vi "KH TURCK ETHERNETIP IOL Diagnostic.vi"(8 "Data_IO":T2, 11 "DataItem.Data":u8[](array[numeric])) -> (3 "Diagnostics":T1)   [LabVIEW 2021]
uses:
  KH TURCK ETHERNETIP TDef Enum IOL Data.ctl
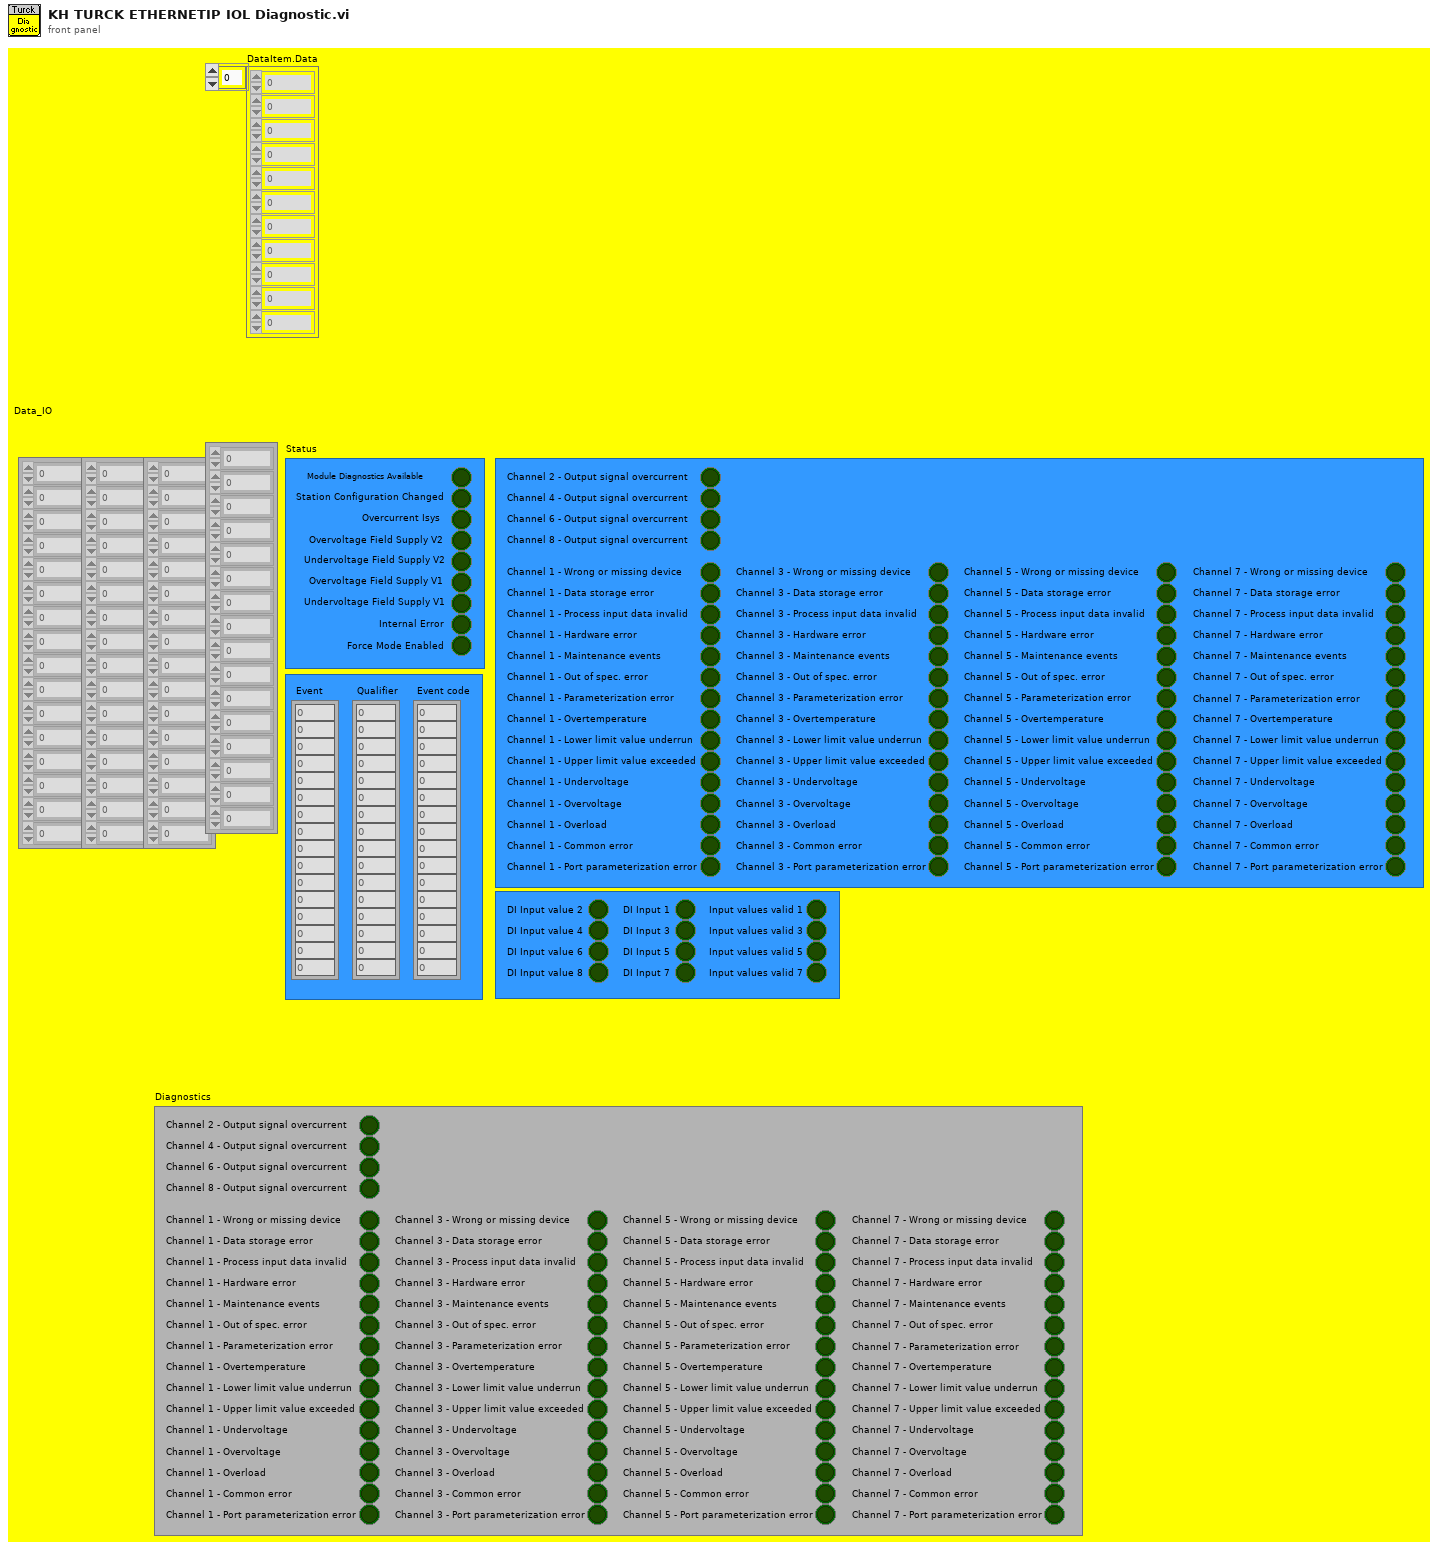
[diagram p1: front panel]
types:
  T1 = cluster{"Channel 2 - Output signal overcurrent":bool, "Channel 4 - Output signal overcurrent":bool, "Channel 6 - Output signal overcurrent":bool, "Channel 8 - Output signal overcurrent":bool, "Channel 1 - Wrong or missing device":bool, "Channel 3 - Wrong or missing device":bool, "Channel 5 - Wrong or missing device":bool, "Channel 7 - Wrong or missing device":bool, "Channel 1 - Data storage error":bool, "Channel 3 - Data storage error":bool, "Channel 5 - Data storage error":bool, "Channel 7 - Data storage error":bool, "Channel 1 - Process input data invalid":bool, "Channel 3 - Process input data invalid":bool, "Channel 5 - Process input data invalid":bool, "Channel 7 - Process input data invalid":bool, "Channel 1 - Hardware error":bool, "Channel 3 - Hardware error":bool, "Channel 5 - Hardware error":bool, "Channel 7 - Hardware error":bool, "Channel 1 - Maintenance events":bool, "Channel 3 - Maintenance events":bool, "Channel 5 - Maintenance events":bool, "Channel 7 - Maintenance events":bool, "Channel 1 - Out of spec. error":bool, "Channel 3 - Out of spec. error":bool, "Channel 5 - Out of spec. error":bool, "Channel 7 - Out of spec. error":bool, "Channel 1 - Parameterization error":bool, "Channel 3 - Parameterization error":bool, "Channel 5 - Parameterization error":bool, "Channel 1 - Overtemperature":bool, "Channel 3 - Overtemperature":bool, "Channel 5 - Overtemperature":bool, "Channel 7 - Overtemperature":bool, "Channel 1 - Lower limit value underrun":bool, "Channel 3 - Lower limit value underrun":bool, "Channel 5 - Lower limit value underrun":bool, "Channel 7 - Lower limit value underrun":bool, "Channel 1 - Upper limit value exceeded":bool, "Channel 3 - Upper limit value exceeded":bool, "Channel 5 - Upper limit value exceeded":bool, "Channel 7 - Upper limit value exceeded":bool, "Channel 1 - Undervoltage":bool, "Channel 3 - Undervoltage":bool, "Channel 5 - Undervoltage":bool, "Channel 7 - Undervoltage":bool, "Channel 1 - Overvoltage":bool, "Channel 3 - Overvoltage":bool, "Channel 5 - Overvoltage":bool, "Channel 7 - Overvoltage":bool, "Channel 1 - Overload":bool, "Channel 3 - Overload":bool, "Channel 5 - Overload":bool, "Channel 7 - Overload":bool, "Channel 1 - Common error":bool, "Channel 3 - Common error":bool, "Channel 5 - Common error":bool, "Channel 7 - Common error":bool, "Channel 1 - Port parameterization error":bool, "Channel 3 - Port parameterization error":bool, "Channel 5 - Port parameterization error":bool, "Channel 7 - Parameterization error":bool, "Channel 7 - Port parameterization error":bool}
  T2 = typedef "KH TURCK ETHERNETIP TDef Enum IOL Data.ctl" = cluster{"Data_Port1":u16[], "Data_Port3":u16[], "Data_Port5":u16[], "Data_Port7":u16[], "Status":cluster{"Undervoltage Field Supply V2":bool, "Overvoltage Field Supply V1":bool, "Undervoltage Field Supply V1":bool, "Internal Error":bool, "Module Diagnostics Available":bool, "Station Configuration Changed":bool, "Overcurrent Isys":bool, "Overvoltage Field Supply V2":bool, "Force Mode Enabled":bool}, "Diagnostics":cluster{"Channel 2 - Output signal overcurrent":bool, "Channel 4 - Output signal overcurrent":bool, "Channel 6 - Output signal overcurrent":bool, "Channel 8 - Output signal overcurrent":bool, "Channel 1 - Wrong or missing device":bool, "Channel 3 - Wrong or missing device":bool, "Channel 5 - Wrong or missing device":bool, "Channel 7 - Wrong or missing device":bool, "Channel 1 - Data storage error":bool, "Channel 3 - Data storage error":bool, "Channel 5 - Data storage error":bool, "Channel 7 - Data storage error":bool, "Channel 1 - Process input data invalid":bool, "Channel 3 - Process input data invalid":bool, "Channel 5 - Process input data invalid":bool, "Channel 7 - Process input data invalid":bool, "Channel 1 - Hardware error":bool, "Channel 3 - Hardware error":bool, "Channel 5 - Hardware error":bool, "Channel 7 - Hardware error":bool, "Channel 1 - Maintenance events":bool, "Channel 3 - Maintenance events":bool, "Channel 5 - Maintenance events":bool, "Channel 7 - Maintenance events":bool, "Channel 1 - Out of spec. error":bool, "Channel 3 - Out of spec. error":bool, "Channel 5 - Out of spec. error":bool, "Channel 7 - Out of spec. error":bool, "Channel 1 - Parameterization error":bool, "Channel 3 - Parameterization error":bool, "Channel 5 - Parameterization error":bool, "Channel 1 - Overtemperature":bool, "Channel 3 - Overtemperature":bool, "Channel 5 - Overtemperature":bool, "Channel 7 - Overtemperature":bool, "Channel 1 - Lower limit value underrun":bool, "Channel 3 - Lower limit value underrun":bool, "Channel 5 - Lower limit value underrun":bool, "Channel 7 - Lower limit value underrun":bool, "Channel 1 - Upper limit value exceeded":bool, "Channel 3 - Upper limit value exceeded":bool, "Channel 5 - Upper limit value exceeded":bool, "Channel 7 - Upper limit value exceeded":bool, "Channel 1 - Undervoltage":bool, "Channel 3 - Undervoltage":bool, "Channel 5 - Undervoltage":bool, "Channel 7 - Undervoltage":bool, "Channel 1 - Overvoltage":bool, "Channel 3 - Overvoltage":bool, "Channel 5 - Overvoltage":bool, "Channel 7 - Overvoltage":bool, "Channel 1 - Overload":bool, "Channel 3 - Overload":bool, "Channel 5 - Overload":bool, "Channel 7 - Overload":bool, "Channel 1 - Common error":bool, "Channel 3 - Common error":bool, "Channel 5 - Common error":bool, "Channel 7 - Common error":bool, "Channel 1 - Port parameterization error":bool, "Channel 3 - Port parameterization error":bool, "Channel 5 - Port parameterization error":bool, "Channel 7 - Parameterization error":bool, "Channel 7 - Port parameterization error":bool}, "Events":cluster{"Event":u8[], "Qualifier":u8[], " Event code":u16[]}, "DXP":cluster{"DI Input value 2":bool, "DI Input value 4":bool, "DI Input value 6":bool, "DI Input value 8":bool, "DI Input 1":bool, "DI Input 3":bool, "DI Input 5":bool, "DI Input 7":bool, "Input values valid 1":bool, "Input values valid 3":bool, "Input values valid 5":bool, "Input values valid 7":bool}}
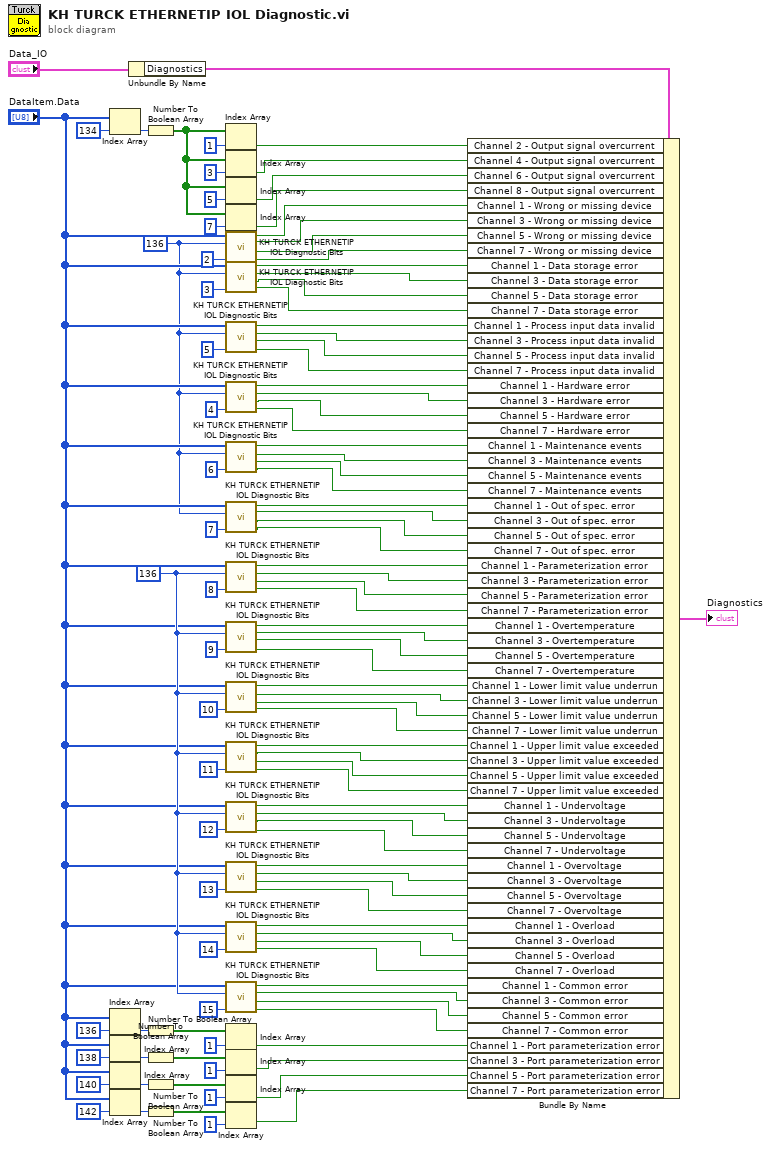
[diagram p0: block diagram]
diagram:
  w32 = 136 ("Start Byte")
  w1 = 136 ("Start Byte")
  n1 = Index Array(array="DataItem.Data", index=134) -> (element=w102:u8)
  n2 = Index Array(array="DataItem.Data", index=136) -> (element=w17:u8)
  n3 = Index Array(array="DataItem.Data", index=138) -> (element=w12:u8)
  n4 = Index Array(array="DataItem.Data", index=140) -> (element=w10:u8)
  n5 = Index Array(array="DataItem.Data", index=142) -> (element=w8:u8)
  n6 = Unbundle By Name("Data_IO") -> ("Diagnostics"=w99:T1)
  n7 = Number To Boolean Array(number=w102) -> (Boolean array=w100:bool[])
  n8 = Number To Boolean Array(number=w17) -> (Boolean array=w23:bool[])
  n9 = Number To Boolean Array(number=w12) -> (Boolean array=w11:bool[])
  n10 = Number To Boolean Array(number=w10) -> (Boolean array=w9:bool[])
  n11 = Number To Boolean Array(number=w8) -> (Boolean array=w7:bool[])
  n12 = Index Array(array=w100, index=1) -> (element=w98:bool)
  n13 = Index Array(array=w100, index=3) -> (element=w97:bool)
  n14 = Index Array(array=w100, index=5) -> (element=w96:bool)
  n15 = Index Array(array=w100, index=7) -> (element=w95:bool)
  n16 = call "KH TURCK ETHERNETIP IOL Diagnostic Bits.vi"("Bit Offset"=2, "Start Byte"=w1, "DataItem.Data"="DataItem.Data") -> ("Bit D"=w87:bool, "Bit C"=w88:bool, "Bit B"=w89:bool, "Bit A"=w90:bool)  [unwired: 5 in]
  n17 = call "KH TURCK ETHERNETIP IOL Diagnostic Bits.vi"("Bit Offset"=3, "Start Byte"=w1, "DataItem.Data"="DataItem.Data") -> ("Bit D"=w83:bool, "Bit C"=w84:bool, "Bit B"=w85:bool, "Bit A"=w86:bool)  [unwired: 5 in]
  n18 = call "KH TURCK ETHERNETIP IOL Diagnostic Bits.vi"("Bit Offset"=5, "Start Byte"=w1, "DataItem.Data"="DataItem.Data") -> ("Bit D"=w79:bool, "Bit C"=w80:bool, "Bit B"=w81:bool, "Bit A"=w82:bool)  [unwired: 5 in]
  n19 = call "KH TURCK ETHERNETIP IOL Diagnostic Bits.vi"("Bit Offset"=4, "Start Byte"=w1, "DataItem.Data"="DataItem.Data") -> ("Bit D"=w75:bool, "Bit C"=w76:bool, "Bit B"=w77:bool, "Bit A"=w78:bool)  [unwired: 5 in]
  n20 = call "KH TURCK ETHERNETIP IOL Diagnostic Bits.vi"("Bit Offset"=6, "Start Byte"=w1, "DataItem.Data"="DataItem.Data") -> ("Bit D"=w70:bool, "Bit C"=w71:bool, "Bit B"=w72:bool, "Bit A"=w73:bool)  [unwired: 5 in]
  n21 = call "KH TURCK ETHERNETIP IOL Diagnostic Bits.vi"("Bit Offset"=7, "Start Byte"=w1, "DataItem.Data"="DataItem.Data") -> ("Bit D"=w65:bool, "Bit C"=w66:bool, "Bit B"=w67:bool, "Bit A"=w68:bool)  [unwired: 5 in]
  n22 = call "KH TURCK ETHERNETIP IOL Diagnostic Bits.vi"("Bit Offset"=8, "Start Byte"=w32, "DataItem.Data"="DataItem.Data") -> ("Bit D"=w60:bool, "Bit C"=w61:bool, "Bit B"=w62:bool, "Bit A"=w63:bool)  [unwired: 5 in]
  n23 = call "KH TURCK ETHERNETIP IOL Diagnostic Bits.vi"("Bit Offset"=9, "Start Byte"=w32, "DataItem.Data"="DataItem.Data") -> ("Bit D"=w55:bool, "Bit C"=w56:bool, "Bit B"=w57:bool, "Bit A"=w58:bool)  [unwired: 5 in]
  n24 = call "KH TURCK ETHERNETIP IOL Diagnostic Bits.vi"("Bit Offset"=10, "Start Byte"=w32, "DataItem.Data"="DataItem.Data") -> ("Bit D"=w50:bool, "Bit C"=w51:bool, "Bit B"=w52:bool, "Bit A"=w53:bool)  [unwired: 5 in]
  n25 = call "KH TURCK ETHERNETIP IOL Diagnostic Bits.vi"("Bit Offset"=11, "Start Byte"=w32, "DataItem.Data"="DataItem.Data") -> ("Bit D"=w45:bool, "Bit C"=w46:bool, "Bit B"=w47:bool, "Bit A"=w48:bool)  [unwired: 5 in]
  n26 = call "KH TURCK ETHERNETIP IOL Diagnostic Bits.vi"("Bit Offset"=12, "Start Byte"=w32, "DataItem.Data"="DataItem.Data") -> ("Bit D"=w40:bool, "Bit C"=w41:bool, "Bit B"=w42:bool, "Bit A"=w43:bool)  [unwired: 5 in]
  n27 = call "KH TURCK ETHERNETIP IOL Diagnostic Bits.vi"("Bit Offset"=13, "Start Byte"=w32, "DataItem.Data"="DataItem.Data") -> ("Bit D"=w35:bool, "Bit C"=w36:bool, "Bit B"=w37:bool, "Bit A"=w38:bool)  [unwired: 5 in]
  n28 = call "KH TURCK ETHERNETIP IOL Diagnostic Bits.vi"("Bit Offset"=14, "Start Byte"=w32, "DataItem.Data"="DataItem.Data") -> ("Bit D"=w28:bool, "Bit C"=w29:bool, "Bit B"=w30:bool, "Bit A"=w31:bool)  [unwired: 5 in]
  n29 = call "KH TURCK ETHERNETIP IOL Diagnostic Bits.vi"("Bit Offset"=15, "Start Byte"=w32, "DataItem.Data"="DataItem.Data") -> ("Bit D"=w24:bool, "Bit C"=w25:bool, "Bit B"=w26:bool, "Bit A"=w27:bool)  [unwired: 5 in]
  n30 = Index Array(array=w23, index=1) -> (element=w6:bool)
  n31 = Index Array(array=w11, index=1) -> (element=w5:bool)
  n32 = Index Array(array=w9, index=1) -> (element=w4:bool)
  n33 = Index Array(array=w7, index=1) -> (element=w3:bool)
  n34 = Bundle By Name(cluster=w99, "Channel 2 - Output signal overcurrent"=w98, "Channel 4 - Output signal overcurrent"=w97, "Channel 6 - Output signal overcurrent"=w96, "Channel 8 - Output signal overcurrent"=w95, "Channel 1 - Wrong or missing device"=w90, "Channel 3 - Wrong or missing device"=w89, "Channel 5 - Wrong or missing device"=w88, "Channel 7 - Wrong or missing device"=w87, "Channel 1 - Data storage error"=w86, "Channel 3 - Data storage error"=w85, "Channel 5 - Data storage error"=w84, "Channel 7 - Data storage error"=w83, "Channel 1 - Process input data invalid"=w82, "Channel 3 - Process input data invalid"=w81, "Channel 5 - Process input data invalid"=w80, "Channel 7 - Process input data invalid"=w79, "Channel 1 - Hardware error"=w78, "Channel 3 - Hardware error"=w77, "Channel 5 - Hardware error"=w76, "Channel 7 - Hardware error"=w75, "Channel 1 - Maintenance events"=w73, "Channel 3 - Maintenance events"=w72, "Channel 5 - Maintenance events"=w71, "Channel 7 - Maintenance events"=w70, "Channel 1 - Out of spec. error"=w68, "Channel 3 - Out of spec. error"=w67, "Channel 5 - Out of spec. error"=w66, "Channel 7 - Out of spec. error"=w65, "Channel 1 - Parameterization error"=w63, "Channel 3 - Parameterization error"=w62, "Channel 5 - Parameterization error"=w61, "Channel 7 - Parameterization error"=w60, "Channel 1 - Overtemperature"=w58, "Channel 3 - Overtemperature"=w57, "Channel 5 - Overtemperature"=w56, "Channel 7 - Overtemperature"=w55, "Channel 1 - Lower limit value underrun"=w53, "Channel 3 - Lower limit value underrun"=w52, "Channel 5 - Lower limit value underrun"=w51, "Channel 7 - Lower limit value underrun"=w50, "Channel 1 - Upper limit value exceeded"=w48, "Channel 3 - Upper limit value exceeded"=w47, "Channel 5 - Upper limit value exceeded"=w46, "Channel 7 - Upper limit value exceeded"=w45, "Channel 1 - Undervoltage"=w43, "Channel 3 - Undervoltage"=w42, "Channel 5 - Undervoltage"=w41, "Channel 7 - Undervoltage"=w40, "Channel 1 - Overvoltage"=w38, "Channel 3 - Overvoltage"=w37, "Channel 5 - Overvoltage"=w36, "Channel 7 - Overvoltage"=w35, "Channel 1 - Overload"=w31, "Channel 3 - Overload"=w30, "Channel 5 - Overload"=w29, "Channel 7 - Overload"=w28, "Channel 1 - Common error"=w27, "Channel 3 - Common error"=w26, "Channel 5 - Common error"=w25, "Channel 7 - Common error"=w24, "Channel 1 - Port parameterization error"=w6, "Channel 3 - Port parameterization error"=w5, "Channel 5 - Port parameterization error"=w4, "Channel 7 - Port parameterization error"=w3) -> (→"Diagnostics":T1)
